vi "AndorCamTempFGV.vi"(8 "error in":errorcluster, 10 "Set_Get":u16(ring) items=["Set", "Get"], 11 "TempIn":i32) -> (0 "error out":errorcluster, 3 "TempOut":i32)   [LabVIEW 2010]
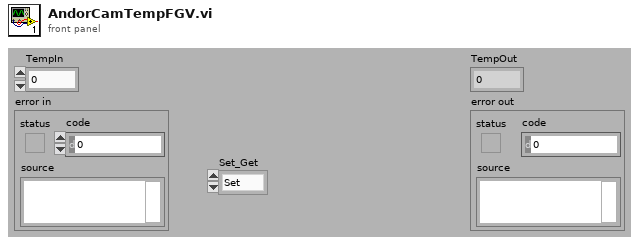
[diagram p1: front panel]
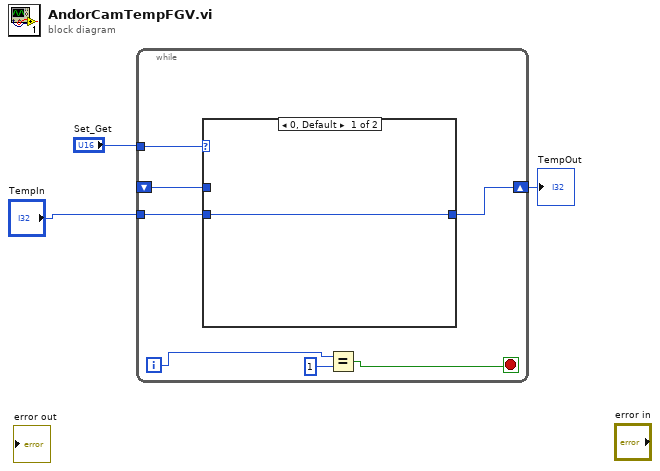
[diagram p0: block diagram]
diagram:
  n1 = while {
    tunnel: "Set_Get" -> [w10]
    tunnel: "TempIn" -> [w9]
    shift-right: [w8] -> w2
    shift-left: _ -> [w7]
    i -> [w4]
    stop <- w5 stop-if-true
    n2 = case shown="0, Default" w10 {
      tunnel: w9 -> [w11 _]
      tunnel: [w11 w12] -> w8
      tunnel: w7 -> [_ w12]
      frame 0, Default {
      }
      frame 1 {
      }
    }
    n3 = Equal?(x=w4, y=1) -> (x = y?=w5:bool)
  }
  "TempOut" <- w2
